vi "Set Revision Number.vi"(9 "Version":string, 11 "Test Executive Builder ViewModel in":refnum<class "Test Executive Builder ViewModel.lvclass">) -> (3 "Test Executive Builder ViewModel out":refnum<class "Test Executive Builder ViewModel.lvclass">)   [LabVIEW 2019, in "Test Executive Builder ViewModel.lvclass"]
uses:
  <vilib>/gpm_packages/@cs/Test-executive-builder/Example/Application/ViewModel/ViewModel/Test Executive Builder ViewModel.lvclass
  <vilib>/gpm_packages/@cs/Test-executive-builder/Example/Application/ViewModel/ViewModel/Test Executive Builder ViewModel.lvclass/Test Executive Builder ViewModel.ctl
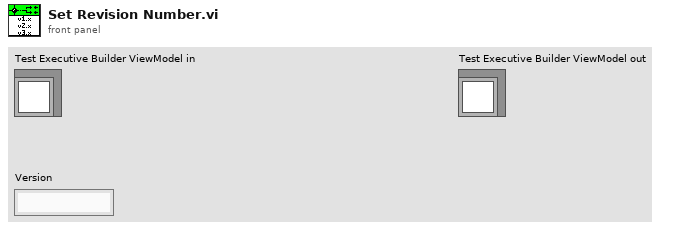
[diagram p1: front panel]
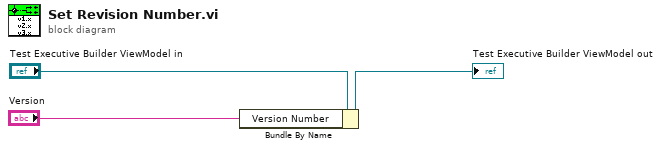
[diagram p0: block diagram]
diagram:
  n1 = Bundle By Name(cluster="Test Executive Builder ViewModel in", "Version Number"="Version") -> (→"Test Executive Builder ViewModel out":refnum<class "Test Executive Builder ViewModel.lvclass">)
